vi "Gestione acq per singola prova.vi"(0 "TIPO COLLEGAMENTO":u16) -> (4 "freddo":cluster{"Visibile ?":bool, "Salva?":bool}[](array[cluster]), 6 "QH":cluster{"Visibile ?":bool, "Salva?":bool}[](array[cluster]), 8 "Termica":cluster{"Visibile ?":bool, "Salva?":bool}[](array[cluster]), 10 "NPSH":cluster{"Visibile ?":bool, "Salva?":bool}[](array[cluster]), 15 "MEI":cluster{"Visibile ?":bool, "Salva?":bool}[](array[cluster]))   [LabVIEW 2019]
uses:
  Global percorso impostazioni.vi
  <vilib>/Utility/file.llb/Read Delimited Spreadsheet (string).vi
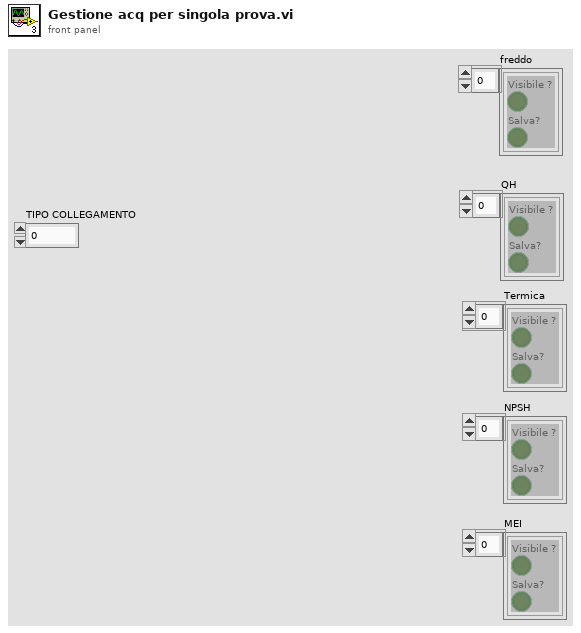
[diagram p1: front panel]
types:
  T1 = cluster{"Nome":string, "QH":cluster{"Visibile ?":bool, "Salva?":bool}, "FREDDO":cluster{"Visibile ?":bool, "Salva?":bool}, "TERMICA":cluster{"Visibile ?":bool, "Salva?":bool}, "NPSH":cluster{"Visibile ?":bool, "Salva?":bool}, "MEI":cluster{"Visibile ?":bool, "Salva?":bool}}
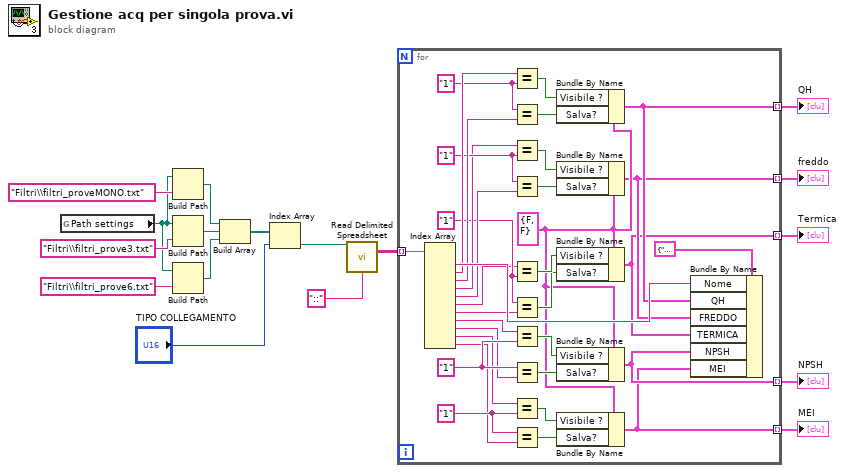
[diagram p0: block diagram]
diagram:
  n1 = global read "Global percorso impostazioni.vi" "Path settings"() -> (w1:path)
  n2 = Build Path(base path=w1, name or relative path="Filtri\\filtri_proveMONO.txt") -> (appended path=w9:path)
  n3 = Build Path(base path=w1, name or relative path="Filtri\\filtri_prove3.txt") -> (appended path=w8:path)
  n4 = Build Path(base path=w1, name or relative path="Filtri\\filtri_prove6.txt") -> (appended path=w7:path)
  n5 = Build Array(w9, w8, w7) -> (w13:path[])
  n6 = Index Array(array=w13, index="TIPO COLLEGAMENTO") -> (element=w15:path)
  n7 = call-poly <vilib>:"Read Delimited Spreadsheet.vi"("file path (dialog if empty)"=w15, "delimiter (\\t)"="::" ("delimiter (\\t)")) -> ("all rows"=w17:string[][])  [unwired: 8 in, 5 out]
  n8 = for {
    tunnel: w17 -> [w50] mode=indexing
    tunnel: [w22] -> w5 mode=indexing
    tunnel: [w21] -> w6 mode=indexing
    tunnel: [w20] -> w4 mode=indexing
    tunnel: [w19] -> w3 mode=indexing
    tunnel: [w18] -> w2 mode=indexing
    w27 = "1" ("y")
    w37 = "1" ("y")
    w36 = "1" ("y")
    w43 = "1" ("y")
    w44 = "1" ("y")
    w25 = cluster{"Visibile ?":bool, "Salva?":bool} {"Visibile ?"=FALSE, "Salva?"=FALSE} ("QH")
    n9 = Index Array(array=w50) -> (element #1=w49:string, element #2=w47:string, element #3=w45:string, element #4=w40:string, element #5=w39:string, element #6=w34:string, element #7=w33:string, element #8=w32:string, element #9=w31:string, element #10=w24:string, element #11=w23:string)  [unwired: 11 in]
    n10 = Equal?(x=w47, y=w44) -> (x = y?=w48:bool)
    n11 = Equal?(x=w44, y=w45) -> (x = y?=w46:bool)
    n12 = Equal?(x=w40, y=w43) -> (x = y?=w41:bool)
    n13 = Equal?(x=w43, y=w39) -> (x = y?=w42:bool)
    n14 = Equal?(x=w34, y=w36) -> (x = y?=w35:bool)
    n15 = Equal?(x=w36, y=w33) -> (x = y?=w30:bool)
    n16 = Equal?(x=w32, y=w37) -> (x = y?=w38:bool)
    n17 = Equal?(x=w37, y=w31) -> (x = y?=w29:bool)
    n18 = Equal?(x=w24, y=w27) -> (x = y?=w26:bool)
    n19 = Equal?(x=w27, y=w23) -> (x = y?=w28:bool)
    n20 = Bundle By Name(cluster=w25, "Visibile ?"=w48, "Salva?"=w46) -> (w22:cluster{"Visibile ?":bool, "Salva?":bool})
    n21 = Bundle By Name(cluster=w25, "Visibile ?"=w41, "Salva?"=w42) -> (w21:cluster{"Visibile ?":bool, "Salva?":bool})
    n22 = Bundle By Name(cluster=w25, "Visibile ?"=w35, "Salva?"=w30) -> (w20:cluster{"Visibile ?":bool, "Salva?":bool})
    n23 = Bundle By Name(cluster=w25, "Visibile ?"=w38, "Salva?"=w29) -> (w19:cluster{"Visibile ?":bool, "Salva?":bool})
    n24 = Bundle By Name(cluster=w25, "Visibile ?"=w26, "Salva?"=w28) -> (w18:cluster{"Visibile ?":bool, "Salva?":bool})
    n25 = Bundle By Name(cluster=T1 {"Nome"="Numero", "QH"={"Visibile ?"=FALSE, "Salva?"=FALSE}, "FREDDO"={"Visibile ?"=FALSE, "Salva?"=FALSE}, "TERMICA"={"Visibile ?"=FALSE, "Salva?"=FALSE}, "NPSH"={"Visibile ?"=FALSE, "Salva?"=FALSE}, "MEI"={"Visibile ?"=FALSE, "Salva?"=FALSE}} ("Cluster"), "Nome"=w49, "QH"=w22, "FREDDO"=w21, "TERMICA"=w20, "NPSH"=w19, "MEI"=w18) -> ()  [unwired: 1 out]
  }
  "freddo" <- w6
  "QH" <- w5
  "Termica" <- w4
  "NPSH" <- w3
  "MEI" <- w2
